vi "stackHorizontally.vi"(4 "spacing[pixel]":u16, 6 "useControlBodyOnly":bool, 7 "verticalAlignment":T1, 8 "error in (no error)":errorcluster, 11 "refs":refnum<vi>[](array[refnum])) -> (0 "error out":errorcluster, 3 "refs(dup)":refnum<vi>[](array[refnum]))   [LabVIEW 2023]
doc: "Arranges the input controls horizontally according to their order in the array, using the specified spacing.\nThe vertical position is processed according to the input 'verticalArrangement'."
uses:
  Ctrls/alignment.ctl
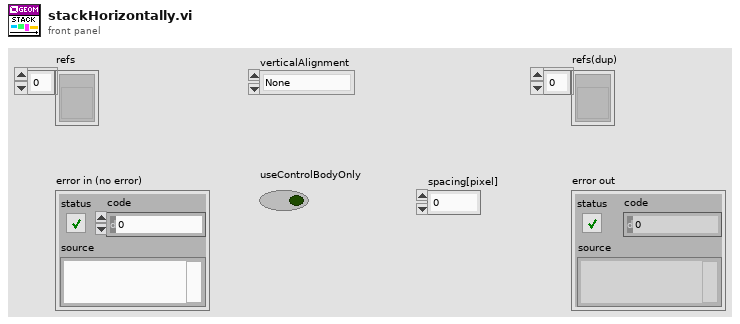
[diagram p1: front panel]
types:
  T1 = typedef "alignment.ctl" = enum16{"None", "AlignTop", "AlignBottom", "AlignHorizontalCenters", "AlignLeft", "AlignRight", "AlignVerticalCenters"}
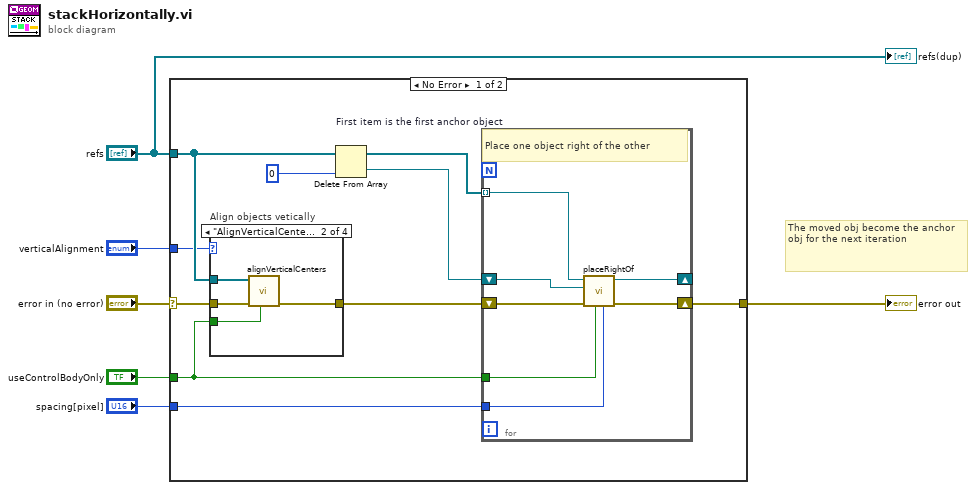
[diagram p0: block diagram]
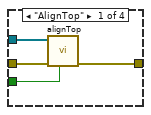
[diagram p2: hidden frame]
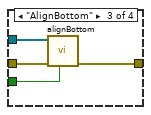
[diagram p3: hidden frame]
diagram:
  # "The moved obj become the anchor obj for the next iteration"
  n1 = case shown="No Error" "error in (no error)" {
    selector: "error in (no error)" -> [w10 w37]
    tunnel: [w16 w37] -> w3
    tunnel: "refs" -> [w11 _]
    tunnel: "useControlBodyOnly" -> [w8 _]
    tunnel: "spacing[pixel]" -> [w12 _]
    tunnel: "verticalAlignment" -> [w7 _]
    frame No Error {
      n2 = case "Align objects vetically" shown="\"AlignVerticalCenters\"" w7 {
        tunnel: w10 -> [w20 w24 w28 w29]
        tunnel: [w19 w23 w27 w29] -> w9
        tunnel: w8 -> [w18 w22 w26 _]
        tunnel: w11 -> [w17 w21 w25 _]
        frame "AlignTop" {
          n3 = call "alignTop.vi"("useControlBodyOnly"=w18, "error in (no error)"=w20, "refs"=w17) -> ("error out"=w19:errorcluster)  [unwired: 7 in, 1 out]
        }
        frame "AlignVerticalCenters" {
          n4 = call "alignVerticalCenters.vi"("useControlBodyOnly"=w22, "error in (no error)"=w24, "refs"=w21) -> ("error out"=w23:errorcluster)  [unwired: 7 in, 1 out]
        }
        frame "AlignBottom" {
          n5 = call "alignBottom.vi"("useControlBodyOnly"=w26, "error in (no error)"=w28, "refs"=w25) -> ("error out"=w27:errorcluster)  [unwired: 7 in, 1 out]
        }
        frame "None", Default {
        }
      }
      n6 = Delete From Array "First item is the first anchor object"(array=w11, index=0) -> (deleted portion=w14:refnum<vi>, array with subset deleted=w13:refnum<vi>[])  [unwired: 1 in]
      n7 = for {
        shift-right: [w35] -> w16
        shift-left: w9 -> [w36]
        tunnel: w13 -> [w31] mode=indexing
        tunnel: w8 -> [w34]
        tunnel: w12 -> [w33]
        shift-right: [w30] -> _
        shift-left: w14 -> [w32]
        # "Place one object right of the other"
        n8 = call "placeRightOf.vi"("spacing[pixel]"=w33, "useControlBodyOnly"=w34, "error in (no error)"=w36, "anchorObject"=w32, "movingObject"=w31) -> ("error out"=w35:errorcluster, "movingObject(dup)"=w30:refnum<vi>)  [unwired: 4 in, 1 out]
      }
    }
    frame Error {
    }
  }
  "error out" <- w3
  "refs(dup)" <- "refs"
